vi "console_panel.vi"() -> ()   [LabVIEW 2014]
doc: "This VI is to serve as a simplified version of the utility_panel.vi, demonstrating primarily the ability to communicate with the connected device via the ASCII commandset.\n\nProduced By:\n\nChristopher Lemieux\nKod Integrations, LLC\n4835 Marianne Drive\nMount Airy, MD 21771\nhttp://www.kodintegrations.com\nemail: clemieux@kodintegrations.com\nphone: (240) 687-1288"
uses:
  common/controls/utility_actions.ctl
  common/controls/commands.ctl
  common/controls/motor_enabled_state_axes_group.ctl
  common/controls/error_actions.ctl
  classes/Controller/_Controller.lvclass
  libraries/common.lvlib
panel:
  in  "help":bool
  out "response":string
  in  "terminate":bool
  in  "raw_cmd":string
  in  "write_cmd":bool
  out "error out":errorcluster
  in  "error in (no error)":errorcluster
  # "COMMAND:"
  # "RESPONSE:"
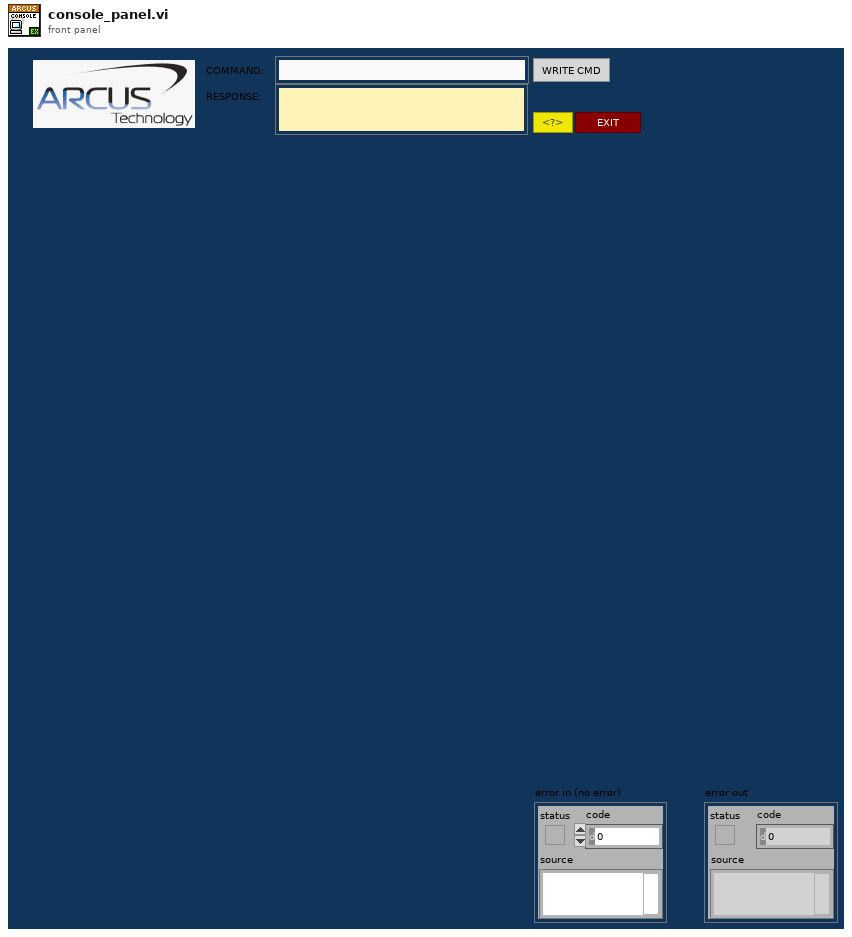
[diagram p1: front panel]
types:
  T1 = typedef "common.lvlib/utility_actions.ctl" = enum16{"------- unused -------", "about", "checkModel", "clearError", "closeRef", "demo", "getAcceleration", "getActualCurrentVal", "getDeviceId", "getDeviceList", "getDigInputs", "getDigOutputs", "getDriverPowerStatus", "getFirmwareVer", "getHighSpeed", "getIdleCurrent", "getLowSpeed", "getMode", "getPolarity", "getPosition", "getProductId", "getRunCurrent", "getStatus", "homeMotorNeg", "homeMotorPos", "initialize", "jogConstNeg", "jogConstPos", "moveToPos", "openRef", "pause", "powerOFF", "powerON", "processEvents", "rawCmd", "setAcceleration", "setDeviceId", "setDigOutput", "setHighSpeed", "setLowSpeed", "setPolarity", "setPosition", "setRunCurrent", "setIdleCurrent", "setMode", "setTimeOuts", "stopImmediately", "stopSlowly", "storeToFlashMem", "updatePanelItems", "validateDemoPos", "validatePos", "waitUntilDone", "zeroPosition"}
  T2 = typedef "common.lvlib/error_actions.ctl" = enum16{"clearBuff", "closeRef", "nodeErr", "noDeviceInfo", "noDevices", "openRef", "sendReceive", "setTimeouts", "unknown"}
  T3 = typedef "common.lvlib/commands.ctl" = enum16{"clear error", "constant jog(-)", "constant jog(+)", "get acceleration", "get actual current", "get device name", "get digital input status", "get digital inputs status", "get digital output status", "get digital outputs status", "get firmware ver", "get high speed", "get idle current", "get low speed", "get micro step", "get motor status", "get move mode", "get polarity", "get position", "get product id", "get power status", "get run current", "get status", "home(-)", "home(+)", "move to position", "power down", "power up", "set acceleration", "set device id", "set digital output", "set digital outputs", "set high speed", "set idle current", "set low speed", "set move mode absolute", "set move mode increment", "set polarity", "set position", "set run current", "stop immediate", "stop slow", "store to memory"}
  T4 = typedef "common.lvlib/motor_enabled_state_axes_group.ctl" = cluster{"x-axis":bool, "y-axis":bool, "z-axis":bool, "u-axis":bool}
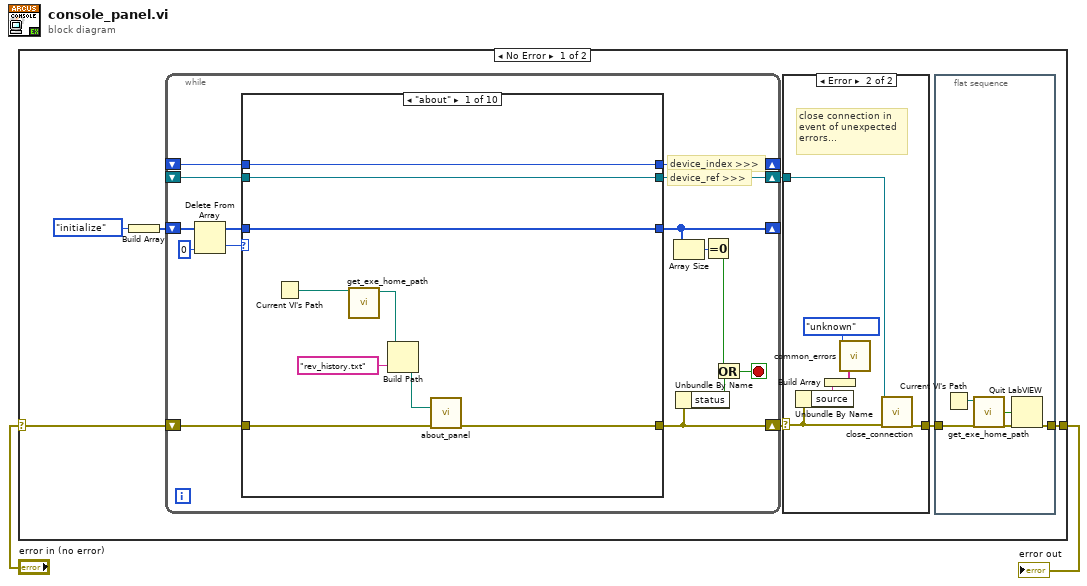
[diagram p0: block diagram]
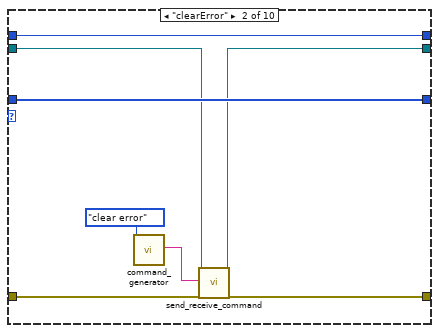
[diagram p3: hidden frame]
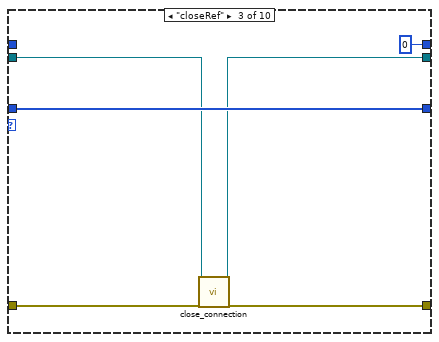
[diagram p4: hidden frame]
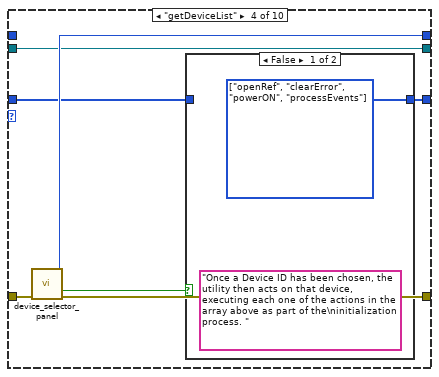
[diagram p5: hidden frame]
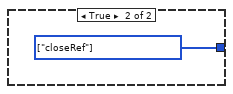
[diagram p6: hidden frame]
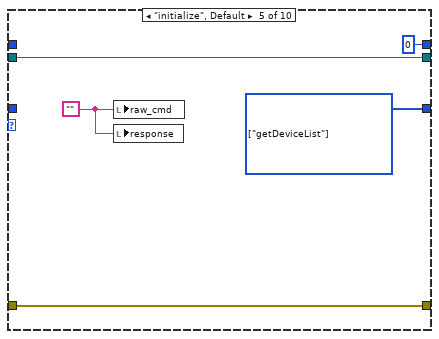
[diagram p7: hidden frame]
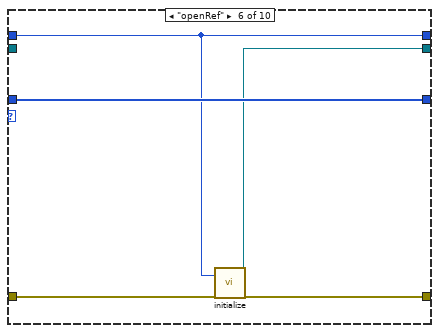
[diagram p8: hidden frame]
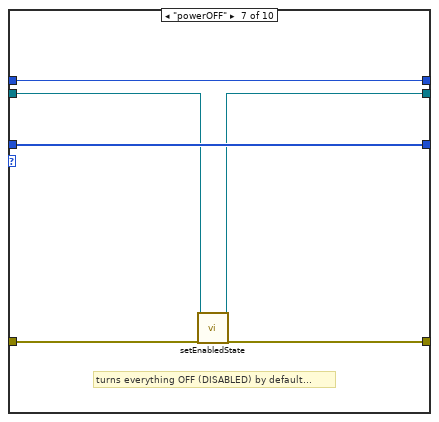
[diagram p9: hidden frame]
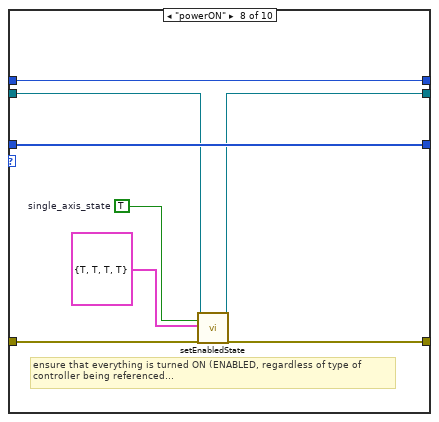
[diagram p10: hidden frame]
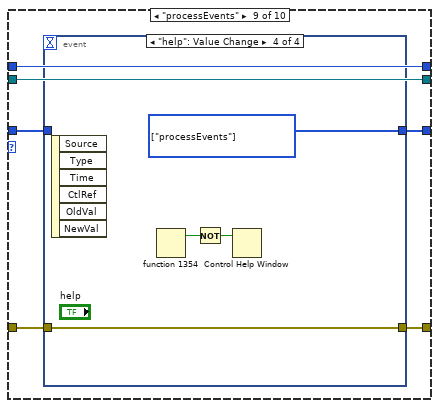
[diagram p11: hidden frame]
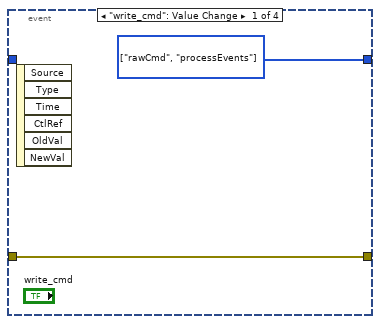
[diagram p12: hidden frame]
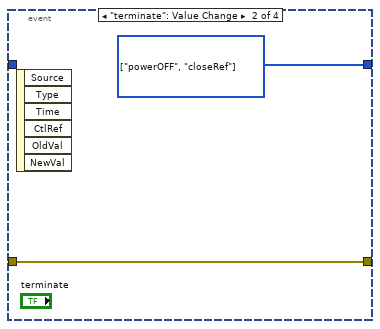
[diagram p13: hidden frame]
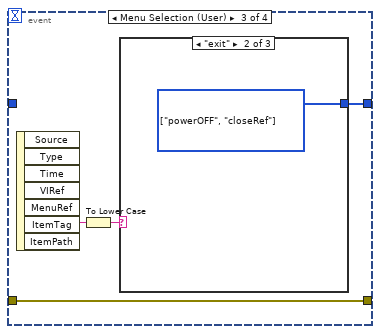
[diagram p14: hidden frame]
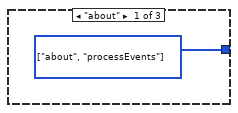
[diagram p15: hidden frame]
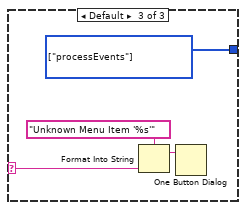
[diagram p16: hidden frame]
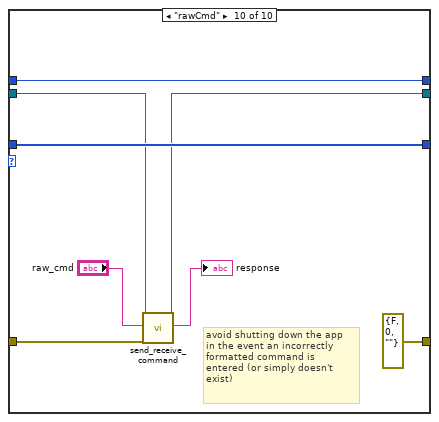
[diagram p17: hidden frame]
diagram:
  n1 = case shown="No Error" "error in (no error)" {
    selector: "error in (no error)" -> [w5 w123]
    tunnel: [w3 w123] -> w1
    frame No Error {
      n2 = Build Array(utility_actions."initialize" ("Enum")) -> (w8:T1[])
      n3 = while {
        shift-right: [w29] -> _
        shift-left: w8 -> [w34]
        shift-right: [w24] -> w7
        shift-left: w5 -> [w30]
        shift-right: [w23] -> w6
        shift-left: _ -> [w22]
        shift-right: [w21] -> _
        shift-left: _ -> [w20]
        stop <- w25 stop-if-true
        # "device_index >>>"
        # "device_ref >>>"
        n4 = Delete From Array(array=w34, index=0) -> (deleted portion=w32:T1, array with subset deleted=w31:T1[])  [unwired: 1 in]
        n5 = case shown="\"about\"" w32 {
          tunnel: w31 -> [w43 w51 w57 w59 _ w76 w82 w90 w93 w121]
          tunnel: [w43 w51 w57 w58 w70 w76 w82 w90 w94 w121] -> w29
          tunnel: w30 -> [w40 w49 w56 w64 w71 w75 w80 w88 w96 w122]
          tunnel: [w39 w48 w55 w63 w71 w74 w79 w87 w95 errorcluster {"status"=FALSE, "code"=0, "source"=""}] -> w24
          tunnel: [w41 w46 w52 w61 w67 w72 w77 w85 w91 w116] -> w23
          tunnel: w22 -> [w41 w47 w53 w61 w67 _ w78 w86 w91 w117]
          tunnel: [w42 w50 0 ("reference (out)") w62 0 ("index") w73 w81 w89 w92 w118] -> w21
          tunnel: w20 -> [w42 w50 _ _ _ w73 w81 w89 w92 w118]
          frame "about" {
            n6 = Current VI's Path() -> (path=w35:path)
            n7 = call "get_exe_home_path.vi"("home_path"=w35) -> ("actual_home_path"=w36:path)  [unwired: 6 in, 1 out]
            n8 = Build Path(base path=w36, name or relative path="rev_history.txt") -> (appended path=w37:path)
            n9 = call "about_panel.vi"("rev_history_filepath"=w37, "error in (no error)"=w40) -> ("error out"=w39:errorcluster)  [unwired: 13 in]
          }
          frame "clearError" {
            n10 = call "command_generator.vi"("cmd (in)"=commands."clear error") -> ("ASCII_cmd (out)"=w44:string)  [unwired: 18 in]
            n11 = call "send_receive_command.vi"("reference (in)"=w47, "ASCII Command (in)"=w44, "error in (no error)"=w49) -> ("reference (out)"=w46:refnum<class "_Controller.lvclass">, "error out"=w48:errorcluster)  [unwired: 12 in, 3 out]
          }
          frame "closeRef" {
            n12 = call "close_connection.vi"("reference (in)"=w53, "error in (no error)"=w56) -> ("reference (out)"=w52:refnum<class "_Controller.lvclass">, "error out"=w55:errorcluster)  [unwired: 16 in]
          }
          frame "getDeviceList" {
            n13 = call "device_selector_panel.vi"("error in (no error)"=w64) -> ("index"=w62:i32, "cancel?"=w60:bool, "error out"=w63:errorcluster)  [unwired: 10 in, 2 out]
            n14 = case shown="False" w60 {
              tunnel: w59 -> [_ _]
              tunnel: [w65 w66] -> w58
              frame False {
                w65 = T1[] [enum."openRef", enum."clearError", enum."powerON", enum."processEvents"] items=["------- unused -------", "about", "checkModel", "clearError", "closeRef", "demo", "getAcceleration", "getActualCurrentVal", "getDeviceId", "getDeviceList", "getDigInputs", "getDigOutputs", "getDriverPowerStatus", "getFirmwareVer", "getHighSpeed", "getIdleCurrent", "getLowSpeed", "getMode", "getPolarity", "getPosition", "getProductId", "getRunCurrent", "getStatus", "homeMotorNeg", "homeMotorPos", "initialize", "jogConstNeg", "jogConstPos", "moveToPos", "openRef", "pause", "powerOFF", "powerON", "processEvents", "rawCmd", "setAcceleration", "setDeviceId", "setDigOutput", "setHighSpeed", "setLowSpeed", "setPolarity", "setPosition", "setRunCurrent", "setIdleCurrent", "setMode", "setTimeOuts", "stopImmediately", "stopSlowly", "storeToFlashMem", "updatePanelItems", "validateDemoPos", "validatePos", "waitUntilDone", "zeroPosition"] ("actions")
                (unwired) "Once a Device ID has been chosen, the utility then acts on that device, executing each one of the actions in the array above as part of the\ninitialization process. "
              }
              frame True {
                w66 = T1[] [enum."closeRef"] items=["------- unused -------", "about", "checkModel", "clearError", "closeRef", "demo", "getAcceleration", "getActualCurrentVal", "getDeviceId", "getDeviceList", "getDigInputs", "getDigOutputs", "getDriverPowerStatus", "getFirmwareVer", "getHighSpeed", "getIdleCurrent", "getLowSpeed", "getMode", "getPolarity", "getPosition", "getProductId", "getRunCurrent", "getStatus", "homeMotorNeg", "homeMotorPos", "initialize", "jogConstNeg", "jogConstPos", "moveToPos", "openRef", "pause", "powerOFF", "powerON", "processEvents", "rawCmd", "setAcceleration", "setDeviceId", "setDigOutput", "setHighSpeed", "setLowSpeed", "setPolarity", "setPosition", "setRunCurrent", "setIdleCurrent", "setMode", "setTimeOuts", "stopImmediately", "stopSlowly", "storeToFlashMem", "updatePanelItems", "validateDemoPos", "validatePos", "waitUntilDone", "zeroPosition"] ("actions")
              }
            }
          }
          frame "initialize", Default {
            w70 = T1[] [enum."getDeviceList"] items=["------- unused -------", "about", "checkModel", "clearError", "closeRef", "demo", "getAcceleration", "getActualCurrentVal", "getDeviceId", "getDeviceList", "getDigInputs", "getDigOutputs", "getDriverPowerStatus", "getFirmwareVer", "getHighSpeed", "getIdleCurrent", "getLowSpeed", "getMode", "getPolarity", "getPosition", "getProductId", "getRunCurrent", "getStatus", "homeMotorNeg", "homeMotorPos", "initialize", "jogConstNeg", "jogConstPos", "moveToPos", "openRef", "pause", "powerOFF", "powerON", "processEvents", "rawCmd", "setAcceleration", "setDeviceId", "setDigOutput", "setHighSpeed", "setLowSpeed", "setPolarity", "setPosition", "setRunCurrent", "setIdleCurrent", "setMode", "setTimeOuts", "stopImmediately", "stopSlowly", "storeToFlashMem", "updatePanelItems", "validateDemoPos", "validatePos", "waitUntilDone", "zeroPosition"] ("actions")
            w68 = ""
            n15 = local write "raw_cmd"(w68) -> ()
            n16 = local write "response"(w68) -> ()
          }
          frame "openRef" {
            n17 = call "initialize.vi"("device_index (in) [0=def]"=w73, "error in (no error)"=w75) -> ("reference (out)"=w72:refnum<class "_Controller.lvclass">, "error out"=w74:errorcluster)  [unwired: 16 in]
          }
          frame "powerOFF" {
            # "turns everything OFF (DISABLED) by default..."
            n18 = call-dynamic "setEnabledState.vi"("Controller in"=w78, "error in (no error)"=w80) -> ("Controller out"=w77:refnum<class "_Controller.lvclass">, "error out"=w79:errorcluster)  [unwired: 14 in, 2 out]
          }
          frame "powerON" {
            w84 = TRUE  # single_axis_state
            # "ensure that everything is turned ON (ENABLED, regardless of type of \ncontroller being referenced..."
            n19 = call-dynamic "setEnabledState.vi"("Controller in"=w86, "state (for single-axis applications only) - (def = DISABLED)"=w84, "axes_states (for multi-axis applications only) - (def = DISABLED)"=T4 {"x-axis"=TRUE, "y-axis"=TRUE, "z-axis"=TRUE, "u-axis"=TRUE}, "error in (no error)"=w88) -> ("Controller out"=w85:refnum<class "_Controller.lvclass">, "error out"=w87:errorcluster)  [unwired: 12 in, 2 out]
          }
          frame "processEvents" {
            n20 = event shown="[3] \"help\": Value Change" {
              selector: _ -> [_ _ _ _]
              dyn-events: _ -> [_ _ _ _]
              timeout: _ -> [_ _ _ _]
              tunnel: [w98 w100 w101 w114] -> w95
              tunnel: w96 -> [w98 w100 w101 w114]
              tunnel: [w97 w99 w102 w113] -> w94
              tunnel: w93 -> [_ _ _ _]
              event "write_cmd": Value Change {
                w97 = T1[] [enum."rawCmd", enum."processEvents"] items=["------- unused -------", "about", "checkModel", "clearError", "closeRef", "demo", "getAcceleration", "getActualCurrentVal", "getDeviceId", "getDeviceList", "getDigInputs", "getDigOutputs", "getDriverPowerStatus", "getFirmwareVer", "getHighSpeed", "getIdleCurrent", "getLowSpeed", "getMode", "getPolarity", "getPosition", "getProductId", "getRunCurrent", "getStatus", "homeMotorNeg", "homeMotorPos", "initialize", "jogConstNeg", "jogConstPos", "moveToPos", "openRef", "pause", "powerOFF", "powerON", "processEvents", "rawCmd", "setAcceleration", "setDeviceId", "setDigOutput", "setHighSpeed", "setLowSpeed", "setPolarity", "setPosition", "setRunCurrent", "setIdleCurrent", "setMode", "setTimeOuts", "stopImmediately", "stopSlowly", "storeToFlashMem", "updatePanelItems", "validateDemoPos", "validatePos", "waitUntilDone", "zeroPosition"] ("actions")
                n21 = event-data() -> ()  [unwired: 1 in, 6 out]
              }
              event "terminate": Value Change {
                w99 = T1[] [enum."powerOFF", enum."closeRef"] items=["------- unused -------", "about", "checkModel", "clearError", "closeRef", "demo", "getAcceleration", "getActualCurrentVal", "getDeviceId", "getDeviceList", "getDigInputs", "getDigOutputs", "getDriverPowerStatus", "getFirmwareVer", "getHighSpeed", "getIdleCurrent", "getLowSpeed", "getMode", "getPolarity", "getPosition", "getProductId", "getRunCurrent", "getStatus", "homeMotorNeg", "homeMotorPos", "initialize", "jogConstNeg", "jogConstPos", "moveToPos", "openRef", "pause", "powerOFF", "powerON", "processEvents", "rawCmd", "setAcceleration", "setDeviceId", "setDigOutput", "setHighSpeed", "setLowSpeed", "setPolarity", "setPosition", "setRunCurrent", "setIdleCurrent", "setMode", "setTimeOuts", "stopImmediately", "stopSlowly", "storeToFlashMem", "updatePanelItems", "validateDemoPos", "validatePos", "waitUntilDone", "zeroPosition"] ("actions")
                n22 = event-data() -> ()  [unwired: 1 in, 6 out]
              }
              event Menu Selection (User) {
                n23 = event-data() -> ("ItemTag"=w104:string)  [unwired: 1 in, 6 out]
                n24 = To Lower Case(string=w104) -> (all lower case string=w103:string)
                n25 = case shown="\"exit\"" w103 {
                  selector: w103 -> [_ _ w107]
                  tunnel: [w105 w106 w110] -> w102
                  frame "about" {
                    w105 = T1[] [enum."about", enum."processEvents"] items=["------- unused -------", "about", "checkModel", "clearError", "closeRef", "demo", "getAcceleration", "getActualCurrentVal", "getDeviceId", "getDeviceList", "getDigInputs", "getDigOutputs", "getDriverPowerStatus", "getFirmwareVer", "getHighSpeed", "getIdleCurrent", "getLowSpeed", "getMode", "getPolarity", "getPosition", "getProductId", "getRunCurrent", "getStatus", "homeMotorNeg", "homeMotorPos", "initialize", "jogConstNeg", "jogConstPos", "moveToPos", "openRef", "pause", "powerOFF", "powerON", "processEvents", "rawCmd", "setAcceleration", "setDeviceId", "setDigOutput", "setHighSpeed", "setLowSpeed", "setPolarity", "setPosition", "setRunCurrent", "setIdleCurrent", "setMode", "setTimeOuts", "stopImmediately", "stopSlowly", "storeToFlashMem", "updatePanelItems", "validateDemoPos", "validatePos", "waitUntilDone", "zeroPosition"] ("actions")
                  }
                  frame "exit" {
                    w106 = T1[] [enum."powerOFF", enum."closeRef"] items=["------- unused -------", "about", "checkModel", "clearError", "closeRef", "demo", "getAcceleration", "getActualCurrentVal", "getDeviceId", "getDeviceList", "getDigInputs", "getDigOutputs", "getDriverPowerStatus", "getFirmwareVer", "getHighSpeed", "getIdleCurrent", "getLowSpeed", "getMode", "getPolarity", "getPosition", "getProductId", "getRunCurrent", "getStatus", "homeMotorNeg", "homeMotorPos", "initialize", "jogConstNeg", "jogConstPos", "moveToPos", "openRef", "pause", "powerOFF", "powerON", "processEvents", "rawCmd", "setAcceleration", "setDeviceId", "setDigOutput", "setHighSpeed", "setLowSpeed", "setPolarity", "setPosition", "setRunCurrent", "setIdleCurrent", "setMode", "setTimeOuts", "stopImmediately", "stopSlowly", "storeToFlashMem", "updatePanelItems", "validateDemoPos", "validatePos", "waitUntilDone", "zeroPosition"] ("actions")
                  }
                  frame Default {
                    w110 = T1[] [enum."processEvents"] items=["------- unused -------", "about", "checkModel", "clearError", "closeRef", "demo", "getAcceleration", "getActualCurrentVal", "getDeviceId", "getDeviceList", "getDigInputs", "getDigOutputs", "getDriverPowerStatus", "getFirmwareVer", "getHighSpeed", "getIdleCurrent", "getLowSpeed", "getMode", "getPolarity", "getPosition", "getProductId", "getRunCurrent", "getStatus", "homeMotorNeg", "homeMotorPos", "initialize", "jogConstNeg", "jogConstPos", "moveToPos", "openRef", "pause", "powerOFF", "powerON", "processEvents", "rawCmd", "setAcceleration", "setDeviceId", "setDigOutput", "setHighSpeed", "setLowSpeed", "setPolarity", "setPosition", "setRunCurrent", "setIdleCurrent", "setMode", "setTimeOuts", "stopImmediately", "stopSlowly", "storeToFlashMem", "updatePanelItems", "validateDemoPos", "validatePos", "waitUntilDone", "zeroPosition"] ("actions")
                    n26 = Format Into String(format string="Unknown Menu Item '%s'" ("message"), w107) -> (resulting string=w108:string)  [unwired: 2 in, 1 out]
                    n27 = One Button Dialog(message=w108) -> ()  [unwired: 1 in, 1 out]
                  }
                }
              }
              event "help": Value Change {
                w113 = T1[] [enum."processEvents"] items=["------- unused -------", "about", "checkModel", "clearError", "closeRef", "demo", "getAcceleration", "getActualCurrentVal", "getDeviceId", "getDeviceList", "getDigInputs", "getDigOutputs", "getDriverPowerStatus", "getFirmwareVer", "getHighSpeed", "getIdleCurrent", "getLowSpeed", "getMode", "getPolarity", "getPosition", "getProductId", "getRunCurrent", "getStatus", "homeMotorNeg", "homeMotorPos", "initialize", "jogConstNeg", "jogConstPos", "moveToPos", "openRef", "pause", "powerOFF", "powerON", "processEvents", "rawCmd", "setAcceleration", "setDeviceId", "setDigOutput", "setHighSpeed", "setLowSpeed", "setPolarity", "setPosition", "setRunCurrent", "setIdleCurrent", "setMode", "setTimeOuts", "stopImmediately", "stopSlowly", "storeToFlashMem", "updatePanelItems", "validateDemoPos", "validatePos", "waitUntilDone", "zeroPosition"] ("actions")
                n28 = event-data() -> ()  [unwired: 1 in, 6 out]
                n29 = fn#1354() -> (1:w112:bool)  [unwired: 1 out]
                n30 = Not(x=w112) -> (.not. x?=w111:bool)
                n31 = Control Help Window(1:w111) -> ()  [unwired: 1 in]
              }
            }
          }
          frame "rawCmd" {
            # "avoid shutting down the app\nin the event an incorrectly\nformatted command is\nentered (or simply doesn't\nexist)"
            n32 = call "send_receive_command.vi"("reference (in)"=w117, "ASCII Command (in)"="raw_cmd", "error in (no error)"=w122) -> ("reference (out)"=w116:refnum<class "_Controller.lvclass">, "response (out)"=→"response":string)  [unwired: 12 in, 3 out]
          }
        }
        n33 = Array Size(array=w29) -> (size(s)=w28:i32)
        n34 = Unbundle By Name(w24) -> ("status"=w26:bool)
        n35 = Equal To 0?(x=w28) -> (x = 0?=w27:bool)
        n36 = Or(x=w27, y=w26) -> (x .or. y?=w25:bool)
      }
      n37 = case shown="Error" w7 {
        selector: w7 -> [w13 w14]
        tunnel: w6 -> [_ w19]
        tunnel: [w13 w18] -> w4
        frame No Error {
        }
        frame Error {
          # "close connection in \nevent of unexpected\nerrors..."
          n38 = Unbundle By Name(w14) -> ("source"=w16:string)
          n39 = Build Array(w16) -> (w15:string[])
          n40 = call "common_errors.vi"("common_errors"=error_actions."unknown" ("errors"), "supp_text"=w15) -> ()  [unwired: 13 in, 1 out]
          n41 = call "close_connection.vi"("reference (in)"=w19, "error in (no error)"=w14) -> ("error out"=w18:errorcluster)  [unwired: 16 in, 1 out]
        }
      }
      n42 = flat-sequence {
        tunnel: w4 -> [w10]
        tunnel: [w10] -> w3
        frame #0 {
          n43 = Current VI's Path() -> (path=w12:path)
          n44 = call "get_exe_home_path.vi"("home_path"=w12) -> ("running in an executable?"=w11:bool)  [unwired: 6 in, 1 out]
          n45 = Quit LabVIEW(quit? (T)=w11) -> ()
        }
      }
    }
    frame Error {
    }
  }
  "error out" <- w1
